vi "OSU110_Connect.vi"(0 "OSU-110":T1(radio), 5 "cmbosu_usb":u16, 7 "txtPort":string caption="Port number(LAN)", 9 "DeviceName":string, 11 "error in (no error)":errorcluster) -> (4 "Reference out":refnum<k24>, 15 "error out":errorcluster)   [LabVIEW 2017]
uses:
  C:/Users/Ssantec_Test/Documents/Instrument_DLL_Sample_Labview_20220902_Ver1.2.2/DLL/x86/InstrumentDLL.dll
  DLL/x86/InstrumentDLL.dll
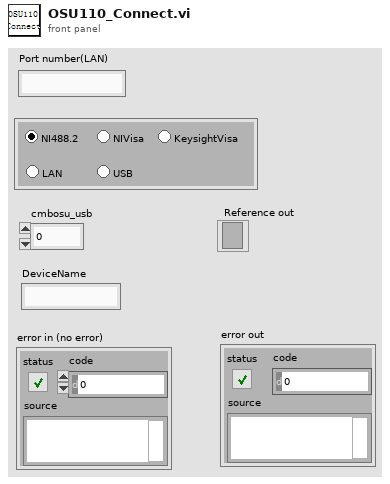
[diagram p1: front panel]
types:
  T1 = enum32{"rdiNI488", "rdiNIvisa", "rdikysightvisa", "rdoLAN", "rdiUSB"}
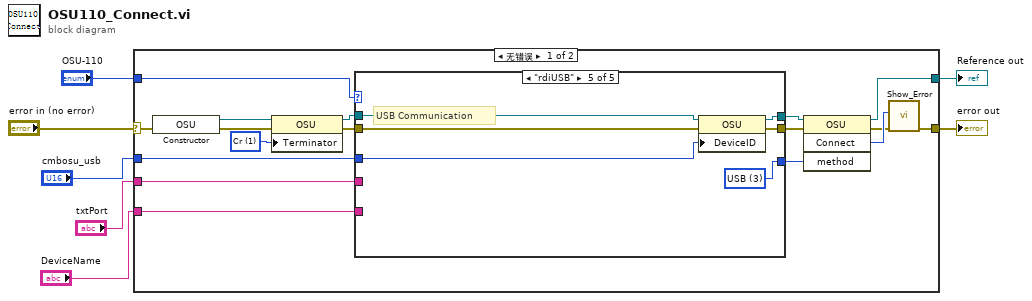
[diagram p0: block diagram]
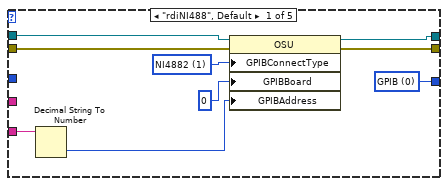
[diagram p2: hidden frame]
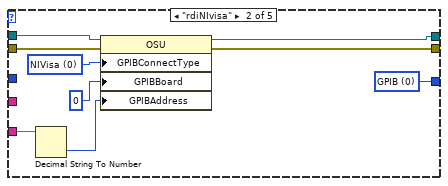
[diagram p3: hidden frame]
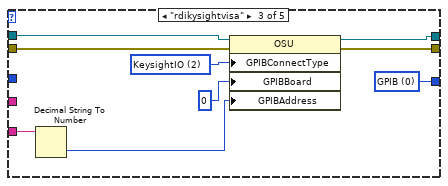
[diagram p4: hidden frame]
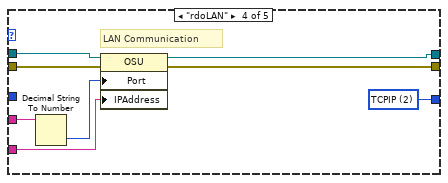
[diagram p5: hidden frame]
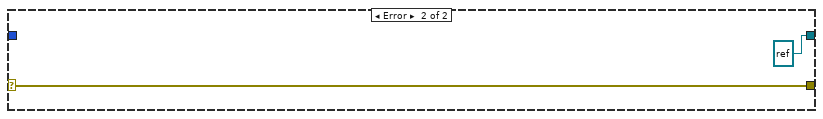
[diagram p6: hidden frame]
diagram:
  n1 = case shown="无错误" "error in (no error)" {
    selector: "error in (no error)" -> [w14 w67]
    tunnel: "DeviceName" -> [w10 _]
    tunnel: [w24 refnum<k24> refnum ("new reference")] -> w6
    tunnel: [w21 w67] -> w4
    tunnel: "OSU-110" -> [w17 _]
    tunnel: "cmbosu_usb" -> [w12 _]
    tunnel: "txtPort" -> [w11 _]
    frame No Error {
      w18 = 1 items=["CrLf", "Cr", "Lf"] ("Terminator")
      n2 = constructor class="OSU"(error in=w14) -> (reference out=w20:refnum<k24>, error out=w19:errorcluster)  [unwired: 2 in, 1 out]
      n3 = property on="属性节点" class="OSU"(reference=w20, error in=w19, "Terminator"=w18) -> (reference out=w16:refnum<k24>, error out=w9:errorcluster)
      n4 = case shown="\"rdiUSB\"" w17 {
        tunnel: w16 -> [w27 w38 w46 w54 w65]
        tunnel: [w28 w36 w47 w58 w64] -> w15
        tunnel: [w33 w39 w48 w59 w63] -> w13
        tunnel: w12 -> [_ _ _ _ w62]
        tunnel: w11 -> [_ _ _ w57 _]
        tunnel: w10 -> [w30 w37 w45 w55 _]
        tunnel: w9 -> [w26 w34 w44 w53 w61]
        tunnel: [w25 w35 w43 w52 w60] -> w8
        frame "rdiNI488", Default {
          w32 = 1 items=["NIVisa", "NI4882", "KeysightIO"] ("GPIBConnectType")
          w33 = 0 items=["GPIB", "C232C", "TCPIP", "USB"] ("method")
          n5 = Decimal String To Number(string=w30) -> (number=w29:i32)  [unwired: 2 in, 1 out]
          n6 = property on="属性节点" class="OSU"(reference=w27, error in=w26, "GPIBConnectType"=w32, "GPIBBoard"=0, "GPIBAddress"=w29) -> (reference out=w28:refnum<k24>, error out=w25:errorcluster)
        }
        frame "rdiNIvisa" {
          w42 = 0 items=["NIVisa", "NI4882", "KeysightIO"] ("GPIBConnectType")
          w39 = 0 items=["GPIB", "C232C", "TCPIP", "USB"] ("method")
          n7 = Decimal String To Number(string=w37) -> (number=w40:i32)  [unwired: 2 in, 1 out]
          n8 = property on="属性节点" class="OSU"(reference=w38, error in=w34, "GPIBConnectType"=w42, "GPIBBoard"=0, "GPIBAddress"=w40) -> (reference out=w36:refnum<k24>, error out=w35:errorcluster)
        }
        frame "rdikysightvisa" {
          w51 = 2 items=["NIVisa", "NI4882", "KeysightIO"] ("GPIBConnectType")
          w48 = 0 items=["GPIB", "C232C", "TCPIP", "USB"] ("method")
          n9 = Decimal String To Number(string=w45) -> (number=w49:i32)  [unwired: 2 in, 1 out]
          n10 = property on="属性节点" class="OSU"(reference=w46, error in=w44, "GPIBConnectType"=w51, "GPIBBoard"=0, "GPIBAddress"=w49) -> (reference out=w47:refnum<k24>, error out=w43:errorcluster)
        }
        frame "rdoLAN" {
          w59 = 2 items=["GPIB", "C232C", "TCPIP", "USB"] ("method")
          # "LAN Communication"
          n11 = Decimal String To Number(string=w57) -> (number=w56:i32)  [unwired: 2 in, 1 out]
          n12 = property on="属性节点" class="OSU"(reference=w54, error in=w53, "Port"=w56, "IPAddress"=w55) -> (reference out=w58:refnum<k24>, error out=w52:errorcluster)
        }
        frame "rdiUSB" {
          w63 = 3 items=["GPIB", "C232C", "TCPIP", "USB"] ("method")
          # "USB Communication"
          n13 = property on="属性节点" class="OSU"(reference=w65, error in=w61, "DeviceID"=w62) -> (reference out=w64:refnum<k24>, error out=w60:errorcluster)
        }
      }
      n14 = invoke on="调用节点" class="OSU" method="Connect"(reference=w15, error in=w8, "method"=w13) -> (reference out=w24:refnum<k24>, error out=w22:errorcluster, "Connect"=w23:i32)  [unwired: 1 in, 1 out]
      n15 = call "Show_Error.vi"("error in (no error)"=w22, "Error"=w23) -> ("error out"=w21:errorcluster)  [unwired: 9 in]
    }
    frame Error {
    }
  }
  "error out" <- w4
  "Reference out" <- w6
